vi "State write value from reference.vi"(8 "error in (no error)":errorcluster, 10 "States":T1, 11 "Data Logger in":refnum<class "Data Logger.lvclass">) -> (0 "error out":errorcluster, 3 "Data Logger out":refnum<class "Data Logger.lvclass">)   [LabVIEW 2013, in "Data Logger.lvlib" / "Data Logger.lvclass"]
uses:
  Data Logger.lvclass
  Display Panel/Abstract Display/Control 1.ctl
  Display Panel/Abstract Display/Abstract Display.lvclass
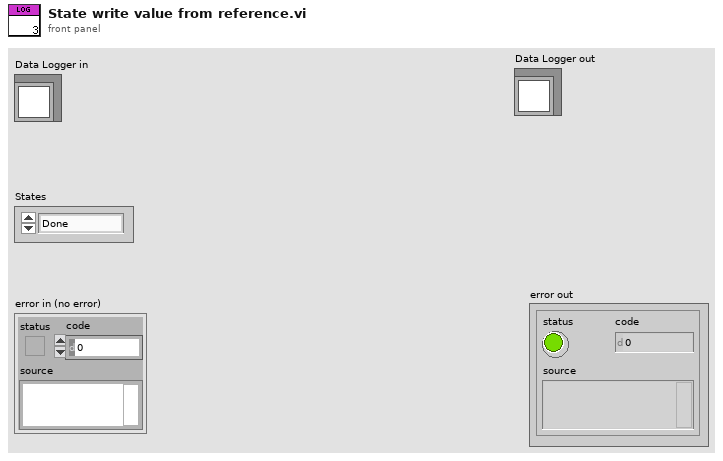
[diagram p1: front panel]
types:
  T1 = typedef "Display Panel.lvlib/Abstract Display.lvclass/Control 1.ctl" = enum16{"Done", "Warming", "Measuring"}
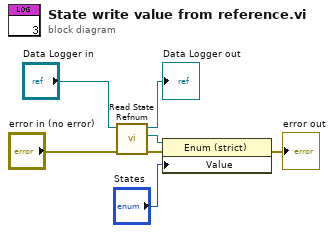
[diagram p0: block diagram]
diagram:
  n1 = call-dynamic "Read State Refnum.vi"("error in (no error)"="error in (no error)", "Data Logger in"="Data Logger in") -> ("error out"=w4:errorcluster, "State Refnum"=w5:refnum<vi>, "Data Logger out"=→"Data Logger out":refnum<class "Data Logger.lvclass">)  [unwired: 7 in]
  n2 = property class="Enum (strict)"(reference=w5, error in=w4, "Value"="States") -> (error out=→"error out":errorcluster)  [unwired: 1 out]
